vi "Write Camera Ini.vi"(0 "ROI":T4={"Global Rectangle"=[0, 0, 640, 480], "Contours"=[{"Contour Type"=0, "ROI Type"=3, "Points"=[4, 4, 636, 476]}]}, 1 "CameraName":string, 5 "Image folder":path, 7 "File Type":T1, 9 "Image Save Rate (s)":dbl=10.0 format="%#_5f", 11 "Record images":bool, 12 "Interface inputs":T3={"Elevation of top of Field of View (cm)"=10.0, "Field of View Height (cm)"=-0.1, "Smooth Length (cm)"=5.0, "Min derivative magnitude"=5.0, "Color Plane"=enum."Green"} {"Smooth Length (cm)" min=0.01 max=1000.0 step=0.1; "Field of View Height (cm)" min=0.1 max=1000.0 step=0.1}, 13 "Rotate":T2) -> ()   [LabVIEW 2015, in "Camera SubVIs.lvlib"]
uses:
  Camera SubVIs.lvlib
  <vilib>/Utility/config.llb/NI_LVConfig.lvlib
  <vilib>/Utility/config.llb/Write Key (String).vi
  <vilib>/Utility/config.llb/Write Key (Double).vi
  <vilib>/Utility/config.llb/Write Key (Path).vi
  <vilib>/Utility/config.llb/Write Key (Boolean).vi
  Calibration and Function folders.ctl
  <vilib>/Utility/config.llb/Write Key (I32).vi
  Interface Inputs.ctl
  Rotate.ctl
  Image File Type.ctl
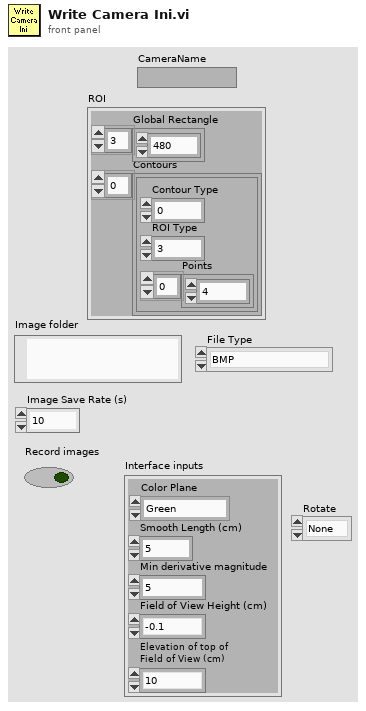
[diagram p1: front panel]
types:
  T1 = typedef "Camera SubVIs.lvlib/Image File Type.ctl" = enum16{"BMP", "JPEG", "JPEG 2000", "PNG", "PNG with Vision Info", "TIFF"}
  T2 = typedef "Camera SubVIs.lvlib/Rotate.ctl" = enum16{"None", "CW", "CCW"}
  T3 = typedef "Camera SubVIs.lvlib/Interface Inputs.ctl" = cluster{"Elevation of top of Field of View (cm)":dbl, "Field of View Height (cm)":dbl, "Smooth Length (cm)":dbl, "Min derivative magnitude":dbl, "Color Plane":enum16{"Red", "Green", "Blue", "Combined"}}
  T4 = cluster{"Global Rectangle":i32[], "Contours":cluster{"Contour Type":u32, "ROI Type":u32, "Points":i32[]}[]}
  T5 = typedef "Calibration and Function folders.ctl" = enum16{"Sensors", "Functions", "Config File", "PublicAppFolder", "New ini File", "Set Config File", "Delete ini File"}
  T6 = typedef "NI_LVConfig.lvlib/Config Data RefNum.ctl" = refnum<k1>
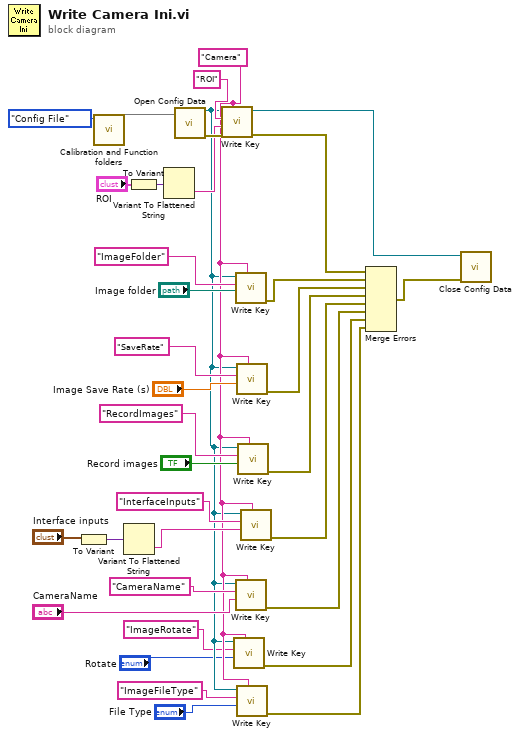
[diagram p0: block diagram]
diagram:
  w8 = "Camera" ("section")
  n1 = To Variant(anything="Interface inputs") -> (Variant=w14:variant)
  n2 = call "Calibration and Function folders.vi"(11:Calibration_and_Function_folders."Config File" ("Folder")) -> (7:w9)  [unwired: 8 in, 2 out]
  n3 = Variant To Flattened String(Variant=w14) -> (data string=w17:string)  [unwired: 1 out]
  n4 = To Variant(anything="ROI") -> (Variant=w33:variant)
  n5 = Variant To Flattened String(Variant=w33) -> (data string=w32:string)  [unwired: 1 out]
  n6 = call <vilib>:"Open Config Data.vi"("configuration file path"=w9) -> ("error out"=w35:errorcluster, "refnum"=w7:T6)  [unwired: 8 in, 1 out]
  n7 = call-poly <vilib>:"Write Key.vi"("section"=w8, "error in (no error)"=w35, "value"=w32, "key"="ROI", "refnum"=w7) -> ("error out"=w22:errorcluster, "refnum out"=w31:T6)  [unwired: 4 in, 1 out]
  n8 = call-poly <vilib>:"Write Key.vi"("section"=w8, "value"="Rotate", "key"="ImageRotate", "refnum"=w7) -> ("error out"=w6:errorcluster)  [unwired: 5 in, 2 out]
  n9 = call-poly <vilib>:"Write Key.vi"("section"=w8, "value"="Image folder", "key"="ImageFolder", "refnum"=w7) -> ("error out"=w21:errorcluster)  [unwired: 5 in, 2 out]
  n10 = call-poly <vilib>:"Write Key.vi"("section"=w8, "value"="CameraName", "key"="CameraName", "refnum"=w7) -> ("error out"=w11:errorcluster)  [unwired: 5 in, 2 out]
  n11 = call-poly <vilib>:"Write Key.vi"("section"=w8, "value"="Image Save Rate (s)", "key"="SaveRate", "refnum"=w7) -> ("error out"=w20:errorcluster)  [unwired: 5 in, 2 out]
  n12 = call-poly <vilib>:"Write Key.vi"("section"=w8, "value"="File Type", "key"="ImageFileType", "refnum"=w7) -> ("error out"=w5:errorcluster)  [unwired: 5 in, 2 out]
  n13 = call-poly <vilib>:"Write Key.vi"("section"=w8, "value"="Record images", "key"="RecordImages", "refnum"=w7) -> ("error out"=w19:errorcluster)  [unwired: 5 in, 2 out]
  n14 = call-poly <vilib>:"Write Key.vi"("section"=w8, "value"=w17, "key"="InterfaceInputs", "refnum"=w7) -> ("error out"=w16:errorcluster)  [unwired: 5 in, 2 out]
  n15 = Merge Errors(w22, w21, w20, w19, w16, w11, w6, w5) -> (w23:errorcluster)
  n16 = call <vilib>:"Close Config Data.vi"("error in (no error)"=w23, "refnum"=w31) -> ()  [unwired: 8 in, 2 out]
